vi "SetMeasurementRegister.vi"(8 "Error In":errorcluster, 9 "Measurement Register":bool[](array[boolean])=[FALSE, FALSE, FALSE, FALSE, FALSE, FALSE, FALSE, FALSE, FALSE, FALSE, FALSE, FALSE, FALSE, FALSE, FALSE], 10 "Program Register":T1, 11 "Keithley 2602 In":refnum<visa-resource-name>) -> (0 "Error Out":errorcluster, 3 "Keithley 2602 Out":refnum<visa-resource-name>)   [LabVIEW 2012, in "Keithley-2602.lvlib"]
uses:
  Keithley-2602.lvlib
  Controls/ProgramRegister.ctl
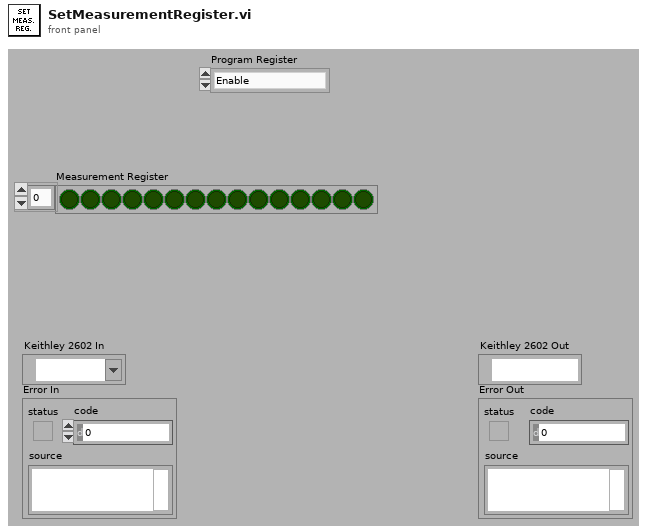
[diagram p1: front panel]
types:
  T1 = typedef "Keithley-2602.lvlib/ProgramRegister.ctl" = enum16{"Enable", "Positive Transition", "Negative Transition"}
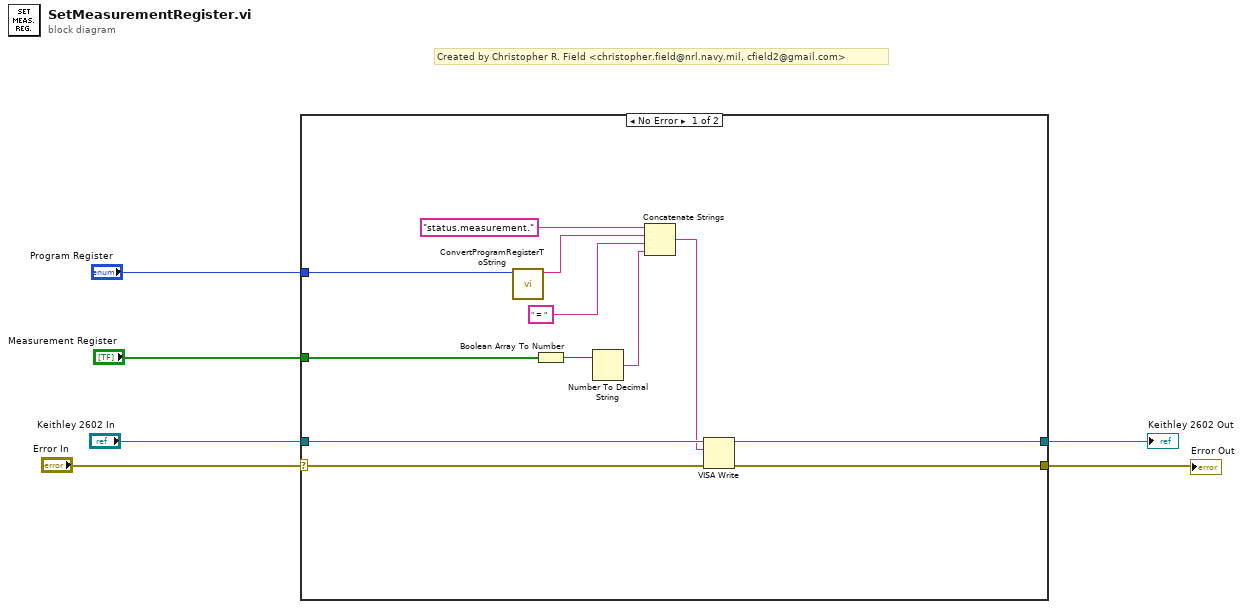
[diagram p0: block diagram]
diagram:
  # "Created by Christopher R. Field <christopher.field@nrl.navy.mil, cfield2@gmail.com>"
  n1 = case shown="No Error" "Error In" {
    selector: "Error In" -> [w7 w19]
    tunnel: "Keithley 2602 In" -> [w18 w20]
    tunnel: [w15 w20] -> w5
    tunnel: [w14 w19] -> w4
    tunnel: "Measurement Register" -> [w13 _]
    tunnel: "Program Register" -> [w8 _]
    frame No Error {
      n2 = call "ConvertProgramRegisterToString.vi"("Program Register"=w8) -> ("Register"=w11:string)  [unwired: 10 in]
      n3 = Boolean Array To Number(Boolean array=w13) -> (number=w17:u32)
      n4 = Number To Decimal String(number=w17) -> (decimal integer string=w9:string)  [unwired: 1 in]
      n5 = Concatenate Strings("status.measurement.", w11, " = " ("string"), w9) -> (w16:string)
      n6 = VISA Write(VISA resource name=w18, write buffer=w16, error in (no error)=w7) -> (VISA resource name out=w15:refnum<visa-resource-name>, error out=w14:errorcluster)  [unwired: 1 out]
    }
    frame Error {
    }
  }
  "Keithley 2602 Out" <- w5
  "Error Out" <- w4
